vi "StopSignal-Generate.vi"(8 "error in (no error)":errorcluster, 10 "reason(\"\")":string, 11 "StopSignal":T1) -> (0 "error out":errorcluster, 3 "StopSignal(dup)":T1)   [LabVIEW 2017, in "StopSignal.lvlib"]
doc: "Generate stop signal."
uses:
  StopSignal.lvlib
  Typedef/StopSignal.ctl
  Typedef/StopReason.ctl
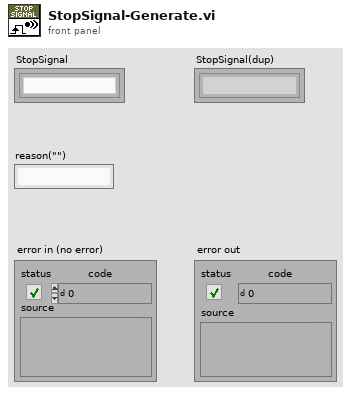
[diagram p1: front panel]
types:
  T1 = typedef "StopSignal.lvlib/StopSignal.ctl" = refnum<k1>
  T2 = typedef "StopSignal.lvlib/StopReason.ctl" = cluster{"Reason":string, "timestamp":timestamp}
  T3 = typedef "StopSignal.lvlib/Def-StopSignalData.ctl" = cluster{"StopEvent":refnum<user-event>, "StopNotifier":refnum<notifier>, "StopReason":T4}
  T4 = typedef "StopSignal.lvlib/def-StopReason.ctl" = cluster{"Reason":string, "timestamp":timestamp}
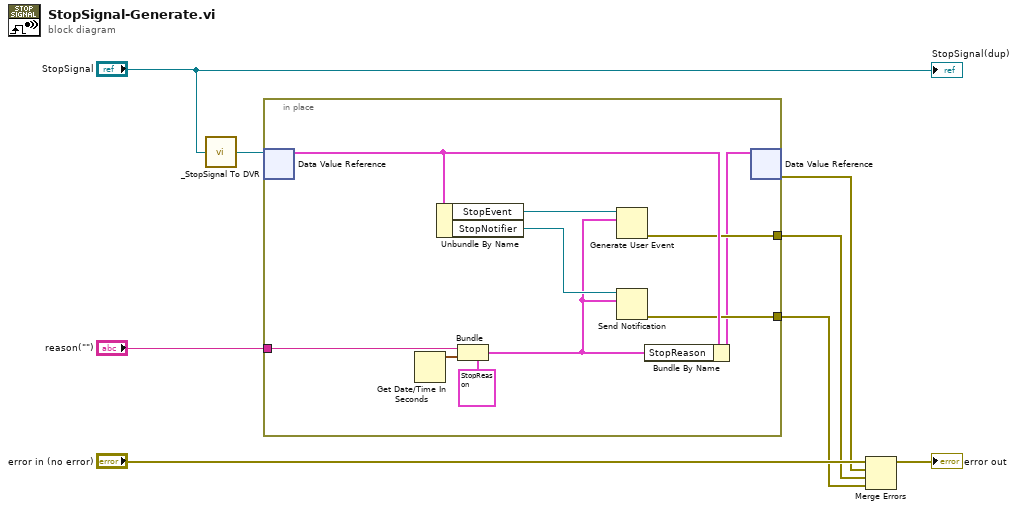
[diagram p0: block diagram]
diagram:
  n1 = call "_StopSignal To DVR.vi"("Refnum in"="StopSignal") -> ("Data Value Reference out"=w6:refnum<data-value>)
  n2 = in-place {
    in-place-border: "reason(\"\")" -> [w12]
    in-place-border: [w15] -> w2
    in-place-border: [w14] -> w1
    n3 = in-place-dvr #1(w6) -> (w18:T3)  [unwired: 1 out]
    n4 = Get Date/Time In Seconds() -> (seconds since 1Jan1904=w11:timestamp)
    n5 = Unbundle By Name(w18) -> ("StopEvent"=w17:refnum<user-event>, "StopNotifier"=w16:refnum<notifier>)
    n6 = Bundle(cluster=T2 {"Reason"="", "timestamp"=timestamp(0 s since 1904-01-01)} ("StopReason"), "Reason"=w12, "timestamp"=w11) -> (w9:T2)
    n7 = Generate User Event(user event=w17, event data cluster=w9) -> (error out=w15:errorcluster)  [unwired: 2 in, 1 out]
    n8 = Send Notification(notification=w9, notifier=w16) -> (error out=w14:errorcluster)  [unwired: 1 in, 1 out]
    n9 = Bundle By Name(cluster=w18, "StopReason"=w9) -> (w10:T3)
    n10 = in-place-dvr #1(w10) -> (w4:errorcluster)  [unwired: 1 out]
  }
  n11 = Merge Errors("error in (no error)", w4, w2, w1) -> (→"error out":errorcluster)
  "StopSignal(dup)" <- "StopSignal"
